vi "Clean Directories.vi"(8 "Error In":errorcluster, 11 "Revert Config":T1={"Revert Paths"={"Archive Path"=path "D:/workspace/revert/todo/todo.zip", "Unzip Directory"=path "D:/workspace/revert/unzip", "Backsave Directory"=path "D:/workspace/revert/backsave", "Output Archive"=path "D:/workspace/revert/backsave", "Backsave Common Directory"=path "D:/workspace/revert/backsave"}, "LabVIEW Files"={"Projects"=[], "Libraries"=[], "Classes"=[], "XControls"=[], "VIs and Controls"=[], "Non LV Files"=[]}, "LabVIEW Version"=enum."8.0"}) -> (0 "Error Out":errorcluster, 3 "Revert Config":T1={"Revert Paths"={"Archive Path"=path "D:/workspace/revert/todo/todo.zip", "Unzip Directory"=path "D:/workspace/revert/unzip", "Backsave Directory"=path "D:/workspace/revert/backsave", "Output Archive"=path "D:/workspace/revert/backsave", "Backsave Common Directory"=path "D:/workspace/revert/backsave"}, "LabVIEW Files"={"Projects"=[], "Libraries"=[], "Classes"=[], "XControls"=[], "VIs and Controls"=[], "Non LV Files"=[]}, "LabVIEW Version"=enum."8.0"})   [LabVIEW 2013, in "LVH-Revert.lvlib"]
uses:
  LVH-Revert.lvlib
  Revert Config.ctl
  Paths.ctl
  LabVIEW Files.ctl
  <vilib>/LabVIEW Hacker/LVH-Toolbox/Common/Private/Type Defs/LabVIEW Version.ctl
  <vilib>/LabVIEW Hacker/LVH-Toolbox/Common/LVH-Common.lvlib
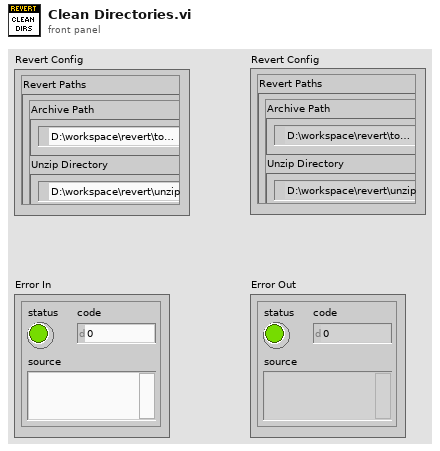
[diagram p1: front panel]
types:
  T1 = typedef "LVH-Revert.lvlib/Revert Config.ctl" = cluster{"Revert Paths":T2, "LabVIEW Files":T3, "LabVIEW Version":T4}
  T2 = typedef "LVH-Revert.lvlib/Paths.ctl" = cluster{"Archive Path":path, "Unzip Directory":path, "Backsave Directory":path, "Output Archive":path, "Backsave Common Directory":path}
  T3 = typedef "LVH-Revert.lvlib/LabVIEW Files.ctl" = cluster{"Projects":path[], "Libraries":path[], "Classes":path[], "XControls":path[], "VIs and Controls":path[], "Non LV Files":path[]}
  T4 = typedef "LVH-Toolbox.lvlib/LVH-Common.lvlib/LabVIEW Version.ctl" = enum16{"8.0", "8.2", "8.6", "9.0", "10.0", "11.0", "12.0", "13.0"}
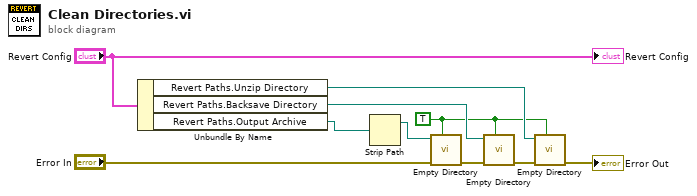
[diagram p0: block diagram]
diagram:
  w1 = TRUE ("Delete Files Without Prompt? (F)")
  n1 = Unbundle By Name("Revert Config") -> ("Revert Paths.Unzip Directory"=w4:path, "Revert Paths.Backsave Directory"=w3:path, "Revert Paths.Output Archive"=w5:path)
  n2 = Strip Path(path=w5) -> (stripped path=w2:path)  [unwired: 1 out]
  n3 = call <vilib>:"Empty Directory.vi"("Delete Files Without Prompt? (F)"=w1, "Error In"="Error In", "Directory"=w2) -> ("Error Out"=w10:errorcluster)  [unwired: 6 in, 2 out]
  n4 = call <vilib>:"Empty Directory.vi"("Delete Files Without Prompt? (F)"=w1, "Error In"=w10, "Directory"=w3) -> ("Error Out"=w8:errorcluster)  [unwired: 6 in, 2 out]
  n5 = call <vilib>:"Empty Directory.vi"("Delete Files Without Prompt? (F)"=w1, "Error In"=w8, "Directory"=w4) -> ("Error Out"=→"Error Out":errorcluster)  [unwired: 6 in, 2 out]
  "Revert Config" <- "Revert Config"
